vi "SP Close Test.vi"(6 "Driver Refs":T2, 7 "Data Source":enum16{"VNA", "Data File"}(ring), 8 "error in (no error)":errorcluster, 11 "Instrument Record":T1) -> (0 "error out":errorcluster {"code" format="%.0x"})   [LabVIEW 2011]
uses:
  TypeDefs/SP Driver Refs.ctl
  drivers/VNA/VNA Driver Ref.ctl
  drivers/SNA/SNA Driver Ref.ctl
  drivers/IMP/IMP Driver Ref.ctl
  server/database/Stations/Instruments/Instrument Record.ctl
  drivers/IMP/IMP Command.ctl
  drivers/VNA/VNA Command.ctl
  drivers/SNA/SNA Command.ctl
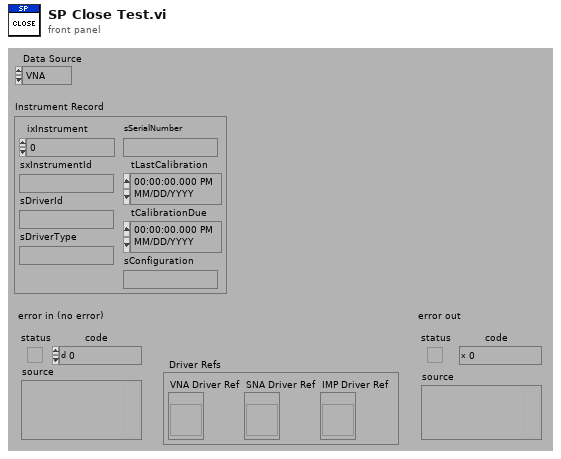
[diagram p1: front panel]
types:
  T1 = typedef "Instrument Record.ctl" = cluster{"ixInstrument":i32, "sxInstrumentId":string, "sDriverId":string, "sDriverType":string, "sSerialNumber":string, "tLastCalibration":timestamp, "tCalibrationDue":timestamp, "sConfiguration":string}
  T2 = typedef "SP Driver Refs.ctl" = cluster{"VNA Driver Ref":T3, "SNA Driver Ref":T4, "IMP Driver Ref":T5}
  T3 = typedef "VNA Driver Ref.ctl" = refnum<vi>
  T4 = typedef "SNA Driver Ref.ctl" = refnum<vi>
  T5 = typedef "IMP Driver Ref.ctl" = refnum<vi>
  T6 = typedef "IMP Command.ctl" = enum16{"LOAD", "INITIALIZE", "IMPORT", "UNLOAD"}
  T7 = typedef "VNA Command.ctl" = enum16{"LOAD", "INITIALIZE", "PRESET", "GET STIMULUS", "SET STIMULUS", "GET CALIBRATION", "CALIBRATE", "RESTORE", "MEASURE", "RELEASE", "UNLOAD", "CONFIRM", "SORT"}
  T8 = typedef "SNA Command.ctl" = enum16{"LOAD", "INITIALIZE", "PRESET", "GET STIMULUS", "SET STIMULUS", "GET CALIBRATION", "CALIBRATE", "RESTORE", "MEASURE", "RELEASE", "UNLOAD", "CONFIRM", "SORT"}
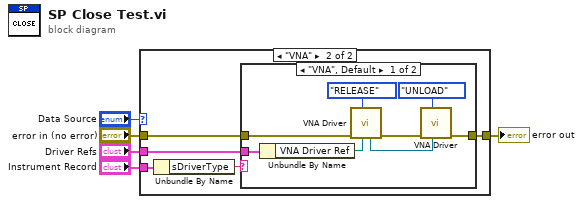
[diagram p0: block diagram]
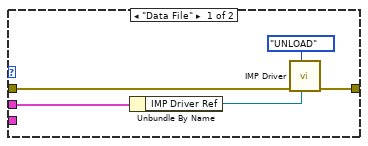
[diagram p2: hidden frame]
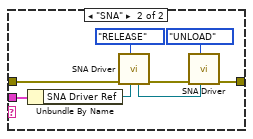
[diagram p3: hidden frame]
diagram:
  n1 = case shown="\"VNA\"" "Data Source" {
    tunnel: "error in (no error)" -> [w9 w15]
    tunnel: "Instrument Record" -> [_ w14]
    tunnel: "Driver Refs" -> [w7 w12]
    tunnel: [w8 w11] -> w2
    frame "Data File" {
      n2 = Unbundle By Name(w7) -> ("IMP Driver Ref"=w6:T5)
      n3 = call "IMP Driver.vi"("Drv Refnum"=w6, "IMP Command"=IMP_Command."UNLOAD" ("VNA Command"), "error in (no error)"=w9) -> ("error out"=w8:errorcluster)  [unwired: 2 in, 6 out]
    }
    frame "VNA" {
      n4 = Unbundle By Name(w14) -> ("sDriverType"=w13:string)
      n5 = case shown="\"VNA\", Default" w13 {
        tunnel: w15 -> [w23 w31]
        tunnel: w12 -> [w21 w29]
        tunnel: [w17 w25] -> w11
        frame "VNA", Default {
          n6 = Unbundle By Name(w21) -> ("VNA Driver Ref"=w20:T3)
          n7 = call "VNA Driver.vi"("Drv Refnum"=w20, "VNA Command"=VNA_Command."RELEASE", "error in (no error)"=w23) -> ("error out"=w18:errorcluster, "dup Drv Refnum"=w16:T3)  [unwired: 4 in, 3 out]
          n8 = call "VNA Driver.vi"("Drv Refnum"=w16, "VNA Command"=VNA_Command."UNLOAD", "error in (no error)"=w18) -> ("error out"=w17:errorcluster)  [unwired: 4 in, 4 out]
        }
        frame "SNA" {
          n9 = Unbundle By Name(w29) -> ("SNA Driver Ref"=w28:T4)
          n10 = call "SNA Driver.vi"("Drv Refnum"=w28, "SNA Command"=SNA_Command."RELEASE", "error in (no error)"=w31) -> ("error out"=w26:errorcluster, "dup Drv Refnum"=w24:T4)  [unwired: 4 in, 3 out]
          n11 = call "SNA Driver.vi"("Drv Refnum"=w24, "SNA Command"=SNA_Command."UNLOAD", "error in (no error)"=w26) -> ("error out"=w25:errorcluster)  [unwired: 4 in, 4 out]
        }
      }
    }
  }
  "error out" <- w2
